vi "Begin.vi"(8 "error in":errorcluster) -> (0 "error out":errorcluster)   [LabVIEW 2017]
doc: "Called before other user functions, this VI is expected to open initial I/O refnums, load in file data, and do all program initialization. Notice that the <B>error out</B> terminal is simply used for data flow. Wiring it to other structures or subVIs ensures that this VI runs first."
uses:
  <vilib>/Rock Robotics/WPI/Joystick/WPI_JoystickDeviceEnum.ctl
  <vilib>/Rock Robotics/WPI/Solenoid/WPI_SolenoidChannel.ctl
  <vilib>/Rock Robotics/SystemInterfaces/DIO/FPGA_DIOPWMChannel.ctl
  <vilib>/Rock Robotics/WPI/DriverStation/WPI_DriverStationRobotMode2.ctl
  <vilib>/Rock Robotics/SystemInterfaces/DIO/FPGA_DIOChannel.ctl
  Robot Global Data.vi
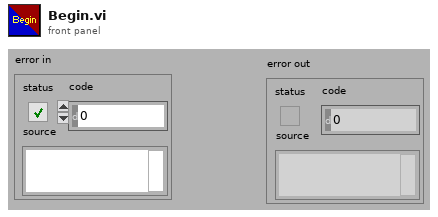
[diagram p1: front panel]
types:
  T1 = typedef "FPGA_DIOChannel.ctl" = enum8{"DIO 0", "DIO 1", "DIO 2", "DIO 3", "DIO 4", "DIO 5", "DIO 6", "DIO 7", "DIO 8", "DIO 9", "DIO MXP 0", "DIO MXP 1", "DIO MXP 2", "DIO MXP 3", "DIO MXP 4", "DIO MXP 5", "DIO MXP 6", "DIO MXP 7", "DIO MXP 8", "DIO MXP 9", "DIO MXP 10", "DIO MXP 11", "DIO MXP 12", "DIO MXP 13", "DIO MXP 14", "DIO MXP 15", "SPI Port CS1", "SPI Port CS2", "SPI Port CS3", "SPI Port MISO", "SPI Port MOSI", "Invalid"}
  T2 = typedef "FPGA_DIOPWMChannel.ctl" = enum8{"PWM 0", "PWM 1", "PWM 2", "PWM 3", "PWM 4", "PWM 5", "PWM 6", "PWM 7", "PWM 8", "PWM 9", "PWM MXP 0", "PWM MXP 1", "PWM MXP 2", "PWM MXP 3", "PWM MXP 4", "PWM MXP 5", "PWM MXP 6", "PWM MXP 7", "PWM MXP 8", "PWM MXP 9", "Invalid"}
  T3 = typedef "WPI_SolenoidChannel.ctl" = enum8{"Solenoid 0", "Solenoid 1", "Solenoid 2", "Solenoid 3", "Solenoid 4", "Solenoid 5", "Solenoid 6", "Solenoid 7", "Invalid"}
  T4 = typedef "WPI_DriverStationRobotMode2.ctl" = enum16{"Autonomous Disabled", "Autonomous Enabled", "Teleop Disabled", "Teleop Enabled", "Disconnected", "Finish", "Test Disabled", "Test Enabled", "Emergency Stopped"}
  T5 = typedef "WPI_JoystickDeviceEnum.ctl" = enum16{"USB 0", "USB 1", "USB 2", "USB 3", "USB 4", "USB 5"}
  T6 = typedef "WPI_MotorControlDeviceRef.ctl" = cluster{"DeviceStatus":errorcluster, "Type":T7, "PWM":cluster{"PWM Channel":T2, "DeadBand":T8}, "CAN":cluster{"Device Number":u8, "SetOutput VI Ref":variant, "GetOutput VI Ref":variant, "Enable VI Ref":variant, "Disable VI Ref":variant, "Data":variant}, "Invert":bool, "DIO PWM":cluster{"PWM \"Enable\" Channel":T2, "DIOChannel":T1, "PWM Rate":dbl}}
  T7 = typedef "WPI_MotorControlType.ctl" = enum16{"PWM", "CAN", "DIO PWM"}
  T8 = typedef "WPI_PWMDeadband.ctl" = cluster{"Name":string, "maxPositivePwm":i32, "minPositivePwm":i32, "centerPwm":i32, "maxNegativePwm":i32, "minNegativePwm":i32, "angularRange":u16}
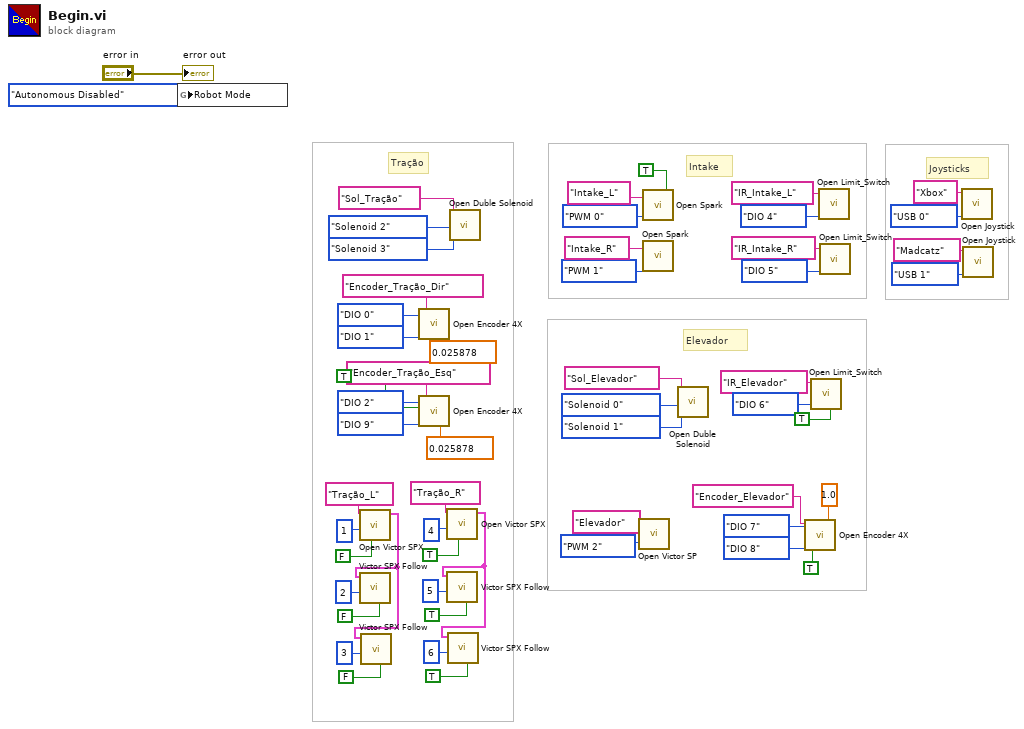
[diagram p0: block diagram]
diagram:
  # "Elevador"
  # "Joysticks"
  # "Tração"
  # "Intake"
  n1 = global write "Robot Global Data.vi" "Robot Mode"(WPI_DriverStationRobotMode2."Autonomous Disabled" ("Robot Mode")) -> ()
  n2 = call "Open Victor SPX.vi"("Invert"=FALSE, "Device Number"=u8 1, "refnum name"="Tração_L") -> ("PhoenixMotorControlDevRef"=w21:T6)  [unwired: 8 in]
  n3 = call "Victor SPX Follow.vi"("Master Controller to Follow"=w21, "Device Number"=u8 2, "Invert"=FALSE) -> ()  [unwired: 7 in]
  n4 = call "Victor SPX Follow.vi"("Master Controller to Follow"=w21, "Device Number"=u8 3, "Invert"=FALSE) -> ()  [unwired: 7 in]
  n5 = call "Open Encoder 4X.vi"("DistancePerCount"=0.025878, "B Channel"=FPGA_DIOChannel."DIO 0", "A Channel"=FPGA_DIOChannel."DIO 1", "refnum name"="Encoder_Tração_Dir") -> ()  [unwired: 2 in]
  n6 = call "Open Encoder 4X.vi"("DistancePerCount"=0.025878, "B Channel"=FPGA_DIOChannel."DIO 2", "A Channel"=FPGA_DIOChannel."DIO 9", "Invert Direction (False)"=TRUE, "refnum name"="Encoder_Tração_Esq") -> ()  [unwired: 1 in]
  n7 = call "Open Victor SPX.vi"("Invert"=TRUE, "Device Number"=u8 4, "refnum name"="Tração_R") -> ("PhoenixMotorControlDevRef"=w13:T6)  [unwired: 8 in]
  n8 = call "Victor SPX Follow.vi"("Master Controller to Follow"=w13, "Device Number"=u8 5, "Invert"=TRUE) -> ()  [unwired: 7 in]
  n9 = call "Victor SPX Follow.vi"("Master Controller to Follow"=w13, "Device Number"=u8 6, "Invert"=TRUE) -> ()  [unwired: 7 in]
  n10 = call "Open Duble Solenoid.vi"("Reverse Solenoid Channel"=WPI_SolenoidChannel."Solenoid 3", "Forward Solenoid Channel"=WPI_SolenoidChannel."Solenoid 2", "refnum name"="Sol_Tração") -> ()  [unwired: 9 in]
  n11 = call "Open Victor SP.vi"("PWM Channel"=FPGA_DIOPWMChannel."PWM 2", "refnum name"="Elevador") -> ()  [unwired: 1 in]
  n12 = call "Open Spark.vi"("Invert"=TRUE, "PWM Channel"=FPGA_DIOPWMChannel."PWM 0", "refnum name"="Intake_L") -> ()
  n13 = call "Open Spark.vi"("PWM Channel"=FPGA_DIOPWMChannel."PWM 1", "refnum name"="Intake_R") -> ()  [unwired: 1 in]
  n14 = call "Open Duble Solenoid.vi"("Reverse Solenoid Channel"=WPI_SolenoidChannel."Solenoid 1", "Forward Solenoid Channel"=WPI_SolenoidChannel."Solenoid 0", "refnum name"="Sol_Elevador") -> ()  [unwired: 9 in]
  n15 = call "Open Encoder 4X.vi"("DistancePerCount"=1.0, "B Channel"=FPGA_DIOChannel."DIO 7", "A Channel"=FPGA_DIOChannel."DIO 8", "Invert Direction (False)"=TRUE, "refnum name"="Encoder_Elevador") -> ()  [unwired: 1 in]
  n16 = call "Open Limit_Switch.vi"("refnum name"="IR_Elevador", "DIO Channel"=FPGA_DIOChannel."DIO 6", "Invert"=TRUE) -> ()  [unwired: 7 in]
  n17 = call "Open Limit_Switch.vi"("refnum name"="IR_Intake_L", "DIO Channel"=FPGA_DIOChannel."DIO 4") -> ()  [unwired: 8 in]
  n18 = call "Open Limit_Switch.vi"("refnum name"="IR_Intake_R", "DIO Channel"=FPGA_DIOChannel."DIO 5") -> ()  [unwired: 8 in]
  n19 = call "Open Joystick.vi"("JoystickDevice"=WPI_JoystickDeviceEnum."USB 0", "refnum name"="Xbox") -> ()  [unwired: 10 in]
  n20 = call "Open Joystick.vi"("JoystickDevice"=WPI_JoystickDeviceEnum."USB 1", "refnum name"="Madcatz") -> ()  [unwired: 10 in]
  "error out" <- "error in"
